vi "Beep.vi"(8 "error in (no error)":errorcluster, 11 "Beep in":refnum<class "Beep.lvclass">) -> (0 "error out":errorcluster, 3 "Beep out":refnum<class "Beep.lvclass">)   [LabVIEW 2016, in "CS++BeepActor.lvlib" / "Beep.lvclass"]
doc: "Generate a beep, either system alert or with user specified frequency and duration."
uses:
  Beep.lvclass
  Beep.lvclass/Beep.ctl
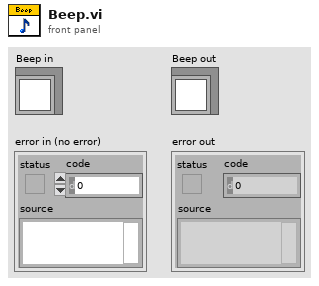
[diagram p1: front panel]
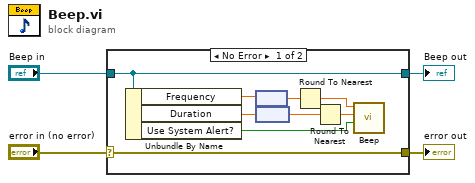
[diagram p0: block diagram]
diagram:
  n1 = case shown="No Error" "error in (no error)" {
    selector: "error in (no error)" -> [w13 w15]
    tunnel: [w13 w15] -> w3
    tunnel: [w12 w14] -> w1
    tunnel: "Beep in" -> [w12 w14]
    frame No Error {
      n2 = Unbundle By Name(w12) -> ("Frequency"=w11:dbl[unit], "Duration"=w10:dbl[unit], "Use System Alert?"=w5:bool)
      n3 = node(w11) -> (w9:dbl)
      n4 = node(w10) -> (w8:dbl)
      n5 = Round To Nearest(number=w9) -> (nearest integer value=w7:dbl)
      n6 = Round To Nearest(number=w8) -> (nearest integer value=w6:dbl)
      n7 = call <vilib>:"Beep.vi"("use system alert? (T)"=w5, "duration (msec)"=w6, "frequency (Hz)"=w7) -> ()  [unwired: 9 in]
    }
    frame Error {
    }
  }
  "error out" <- w3
  "Beep out" <- w1
